vi "save_data_mt_connect (SubVI).vi"(0 "Byte Stream File in":refnum<file>, 1 "Array 2":string[](array[string]), 2 "Array":dbl[](array[numeric]), 3 "current time":timestamp, 5 "base path":path, 7 "Record  SS 661":bool, 9 "Boolean 3":bool, 11 "error in (no error)":errorcluster) -> (4 "Byte Stream File out":refnum<file>, 6 "Boolean 2":bool, 15 "error out":errorcluster)   [LabVIEW 2014]
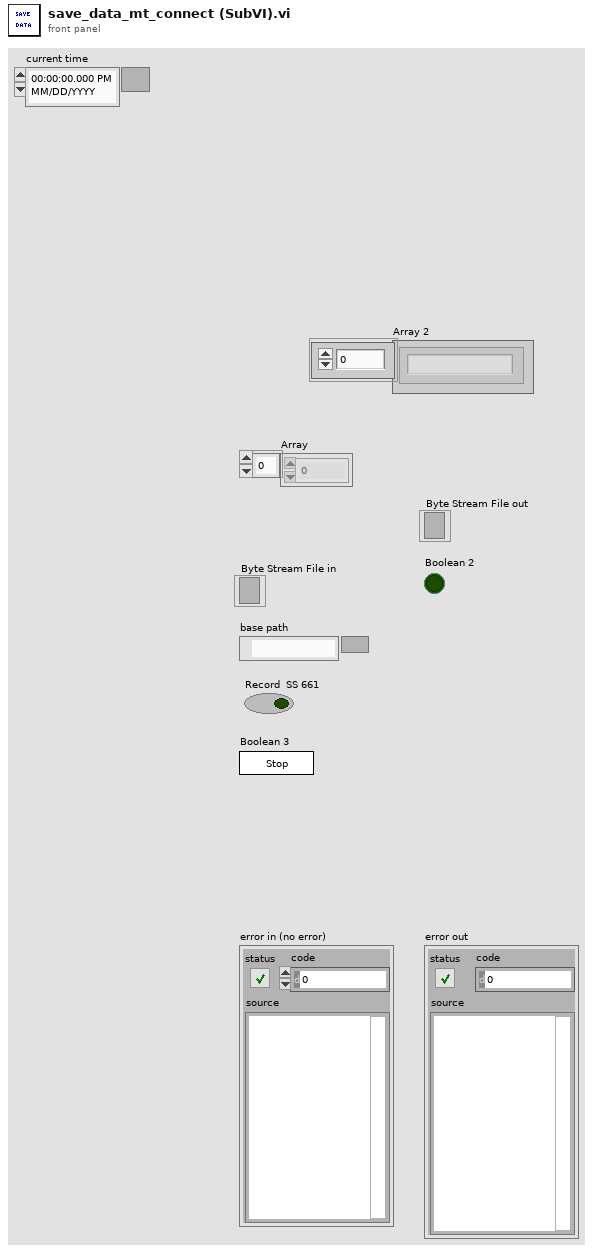
[diagram p1: front panel]
types:
  T1 = enum16{"NotSaving", "Create", "Reading", "Closing"}
  T2 = enum16{"open", "replace", "create", "open or create", "replace or create", "replace or create with confirmation"}
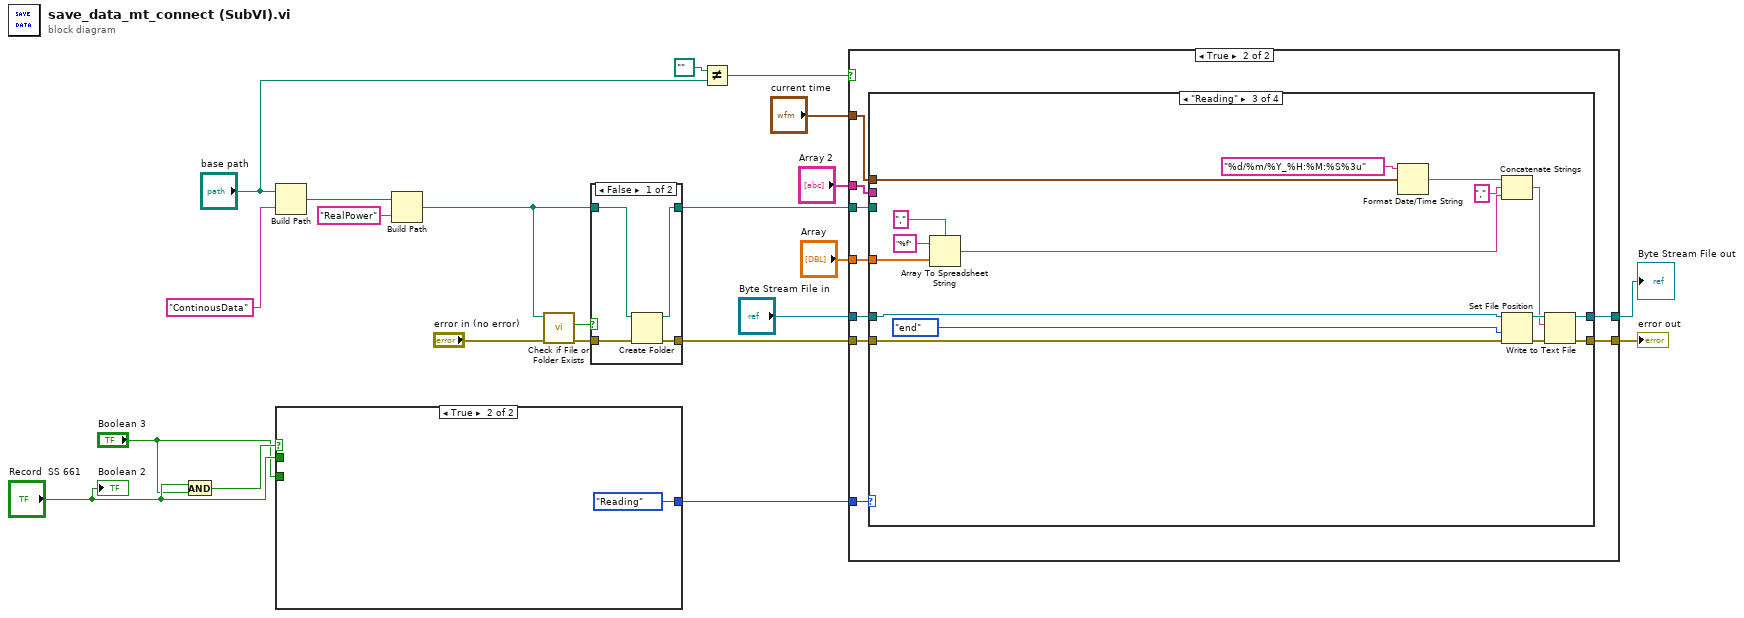
[diagram p0: block diagram]
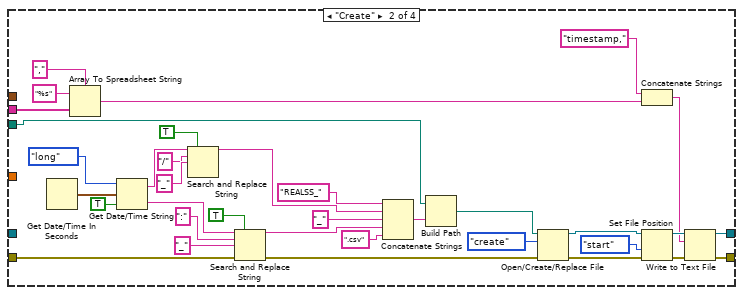
[diagram p5: hidden frame]
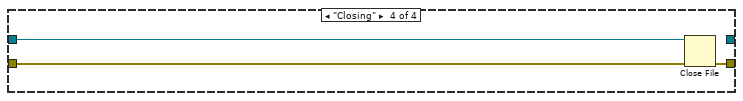
[diagram p6: hidden frame]
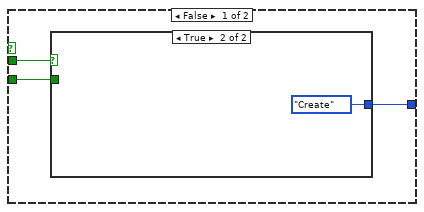
[diagram p7: hidden frame]
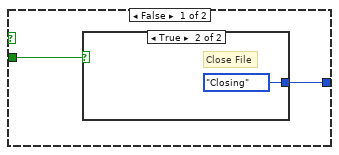
[diagram p8: hidden frame]
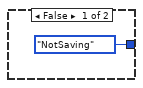
[diagram p9: hidden frame]
diagram:
  n1 = And(x="Record  SS 661", y="Boolean 3") -> (x .and. y?=w17:bool)
  n2 = Build Path(base path="base path", name or relative path="ContinousData") -> (appended path=w8:path)
  n3 = case shown="True" w17 {
    tunnel: "Boolean 3" -> [w25 _]
    tunnel: [w24 T1."Reading" ("Enum")] -> w16
    tunnel: "Record  SS 661" -> [w23 _]
    frame False {
      n4 = case shown="True" w23 {
        tunnel: w25 -> [w27 _]
        tunnel: [w26 T1."Create" ("Enum")] -> w24
        frame False {
          n5 = case shown="True" w27 {
            tunnel: [T1."NotSaving" ("Enum") T1."Closing" ("Enum")] -> w26
            frame False {
            }
            frame True {
              # "Close File"
            }
          }
        }
        frame True {
        }
      }
    }
    frame True {
    }
  }
  n6 = Build Path(base path=w8, name or relative path="RealPower") -> (appended path=w7:path)
  n7 = call <vilib>:"Check if File or Folder Exists.vi"("error in (no error)"="error in (no error)", "path"=w7) -> ("error out"=w10:errorcluster, "file or folder exists?"=w11:bool)  [unwired: 7 in, 1 out]
  n8 = case shown="False" w11 {
    tunnel: [w35 w37] -> w5
    tunnel: w10 -> [w34 w37]
    tunnel: w7 -> [w33 w36]
    tunnel: [w32 w36] -> w6
    frame False {
      n9 = Create Folder(path (use dialog)=w33, error in=w34) -> (created path=w32:path, error out=w35:errorcluster)  [unwired: 1 in, 1 out]
    }
    frame True {
    }
  }
  n10 = Not Equal?(x=path "" ("Project Folder"), y="base path") -> (x != y?=w12:bool)
  n11 = case shown="True" w12 {
    tunnel: w6 -> [_ w45]
    tunnel: "Array" -> [_ w47]
    tunnel: w16 -> [_ w46]
    tunnel: w5 -> [w38 w44]
    tunnel: "Byte Stream File in" -> [_ w43]
    tunnel: [_ w42] -> w21
    tunnel: [w38 w41] -> w15
    tunnel: "Array 2" -> [_ w40]
    tunnel: "current time" -> [_ w39]
    frame False {
    }
    frame True {
      n12 = case shown="\"Reading\"" w46 {
        tunnel: w47 -> [_ _ w93 _]
        tunnel: w45 -> [_ w84 _ _]
        tunnel: w44 -> [w49 w65 w96 w103]
        tunnel: w43 -> [w48 _ w99 w101]
        tunnel: [w48 w57 w94 _] -> w42
        tunnel: [w49 w56 w95 w102] -> w41
        tunnel: w40 -> [_ w53 _ _]
        tunnel: w39 -> [_ _ w85 _]
        frame "NotSaving", Default {
        }
        frame "Create" {
          n13 = Get Date/Time In Seconds() -> (seconds since 1Jan1904=w81:timestamp)
          n14 = Array To Spreadsheet String(delimiter (Tab)=",", array=w53, 3:"%s" ("format string")) -> (spreadsheet string=w51:string)
          n15 = Get Date/Time String(date format (0)=enum16{"short", "long", "abbreviated"}."long", seconds (now)=w81, want seconds? (F)=TRUE) -> (date string=w79:string, time string=w75:string)
          n16 = Search and Replace String(replace all?=TRUE ("replace all? (F)"), input string=w79, search string="/", replace string="_" ("replace string (\"\")")) -> (result string=w72:string)  [unwired: 4 in, 3 out]
          n17 = Search and Replace String(replace all?=TRUE ("replace all? (F)"), input string=w75, search string=":", replace string="_" ("replace string (\"\")"), error in=w65) -> (result string=w70:string, error out=w66:errorcluster)  [unwired: 3 in, 2 out]
          n18 = Concatenate Strings("REALSS_" ("string"), w72, "_" ("string"), w70, ".csv" ("string")) -> (w68:string)
          n19 = Build Path(base path=w84, name or relative path=w68) -> (appended path=w83:path)
          n20 = Open/Create/Replace File(file path (use dialog)=w83, error in=w66, operation (0:open)=T2."create") -> (refnum out=w62:refnum<file>, error out=w61:errorcluster)  [unwired: 3 in, 1 out]
          n21 = Concatenate Strings("timestamp," ("string"), w51) -> (w50:string)
          n22 = Set File Position(refnum=w62, from (0:start)=enum16{"start", "end", "current"}."start", error in=w61) -> (refnum out=w58:refnum<file>, error out=w59:errorcluster)  [unwired: 1 in]
          n23 = Write to Text File(file (use dialog)=w58, text=w50, error in=w59) -> (refnum out=w57:refnum<file>, error out=w56:errorcluster)  [unwired: 1 in, 1 out]
        }
        frame "Reading" {
          n24 = Array To Spreadsheet String(delimiter (Tab)=",", array=w93, 3:"%f" ("format string")) -> (spreadsheet string=w87:string)
          n25 = Format Date/Time String(time format string (%c)="%d/%m/%Y_%H:%M:%S%3u", seconds (now)=w85) -> (date/time string=w90:string)  [unwired: 1 in]
          n26 = Concatenate Strings(w90, "," ("string"), w87) -> (w89:string)
          n27 = Set File Position(refnum=w99, from (0:start)=enum16{"start", "end", "current"}."end", error in=w96) -> (refnum out=w98:refnum<file>, error out=w97:errorcluster)  [unwired: 1 in]
          n28 = Write to Text File(file (use dialog)=w98, text=w89, error in=w97) -> (refnum out=w94:refnum<file>, error out=w95:errorcluster)  [unwired: 1 in, 1 out]
        }
        frame "Closing" {
          n29 = Close File(refnum=w101, error in=w103) -> (error out=w102:errorcluster)  [unwired: 1 out]
        }
      }
    }
  }
  "error out" <- w15
  "Byte Stream File out" <- w21
  "Boolean 2" <- "Record  SS 661"
